vi "AppendListOfSubVIsToReport_Mutation.vi"(0 "Diagram":refnum<vi>, 5 "ObjRef":refnum<vi>, 6 "Kind":string="SubVI", 7 "Information":string="<Not A Path>") -> (3 "Replace?":bool)   [LabVIEW 2020]
uses:
  <vilib>/Utility/Data Type/NI_Data Type.lvlib
  <vilib>/Utility/Data Type/Type Definitions/Data Type.ctl
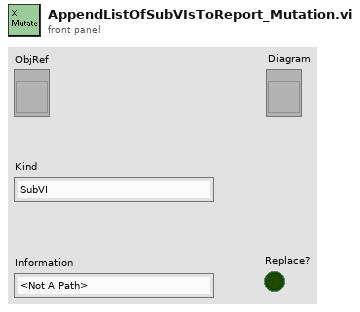
[diagram p1: front panel]
types:
  T1 = typedef "NI_Data Type.lvlib/Data Type.ctl" = enum8{"Invalid Type", "Void", "I8", "I16", "I32", "I64", "U8", "U16", "U32", "U64", "Single Float", "Double Float", "Extended Float", "Single Complex", "Double Complex", "Extended Complex", "Enum U8", "Enum U16", "Enum U32", "Enum U64", "Single Float With Unit", "Double Float With Unit", "Extended Float With Unit", "Single Complex with Unit", "Double Complex with Unit", "Extended Complex with Unit", "Boolean", "String", "Path", "Picture", "Tag", "Array", "Cluster", "Variant", "LV Variant", "Waveform", "Timestamp", "Digital Waveform", "Digital Data", "ExpressData", "Refnum", "External Data", "VI", "Poly VI", "LabVIEW Class Instance", "Fixed Point", "Set Collection", "Map Collection"}
  T2 = typedef "LVPositionTypeDef.ctl" = cluster{"Left":i32, "Top":i32}
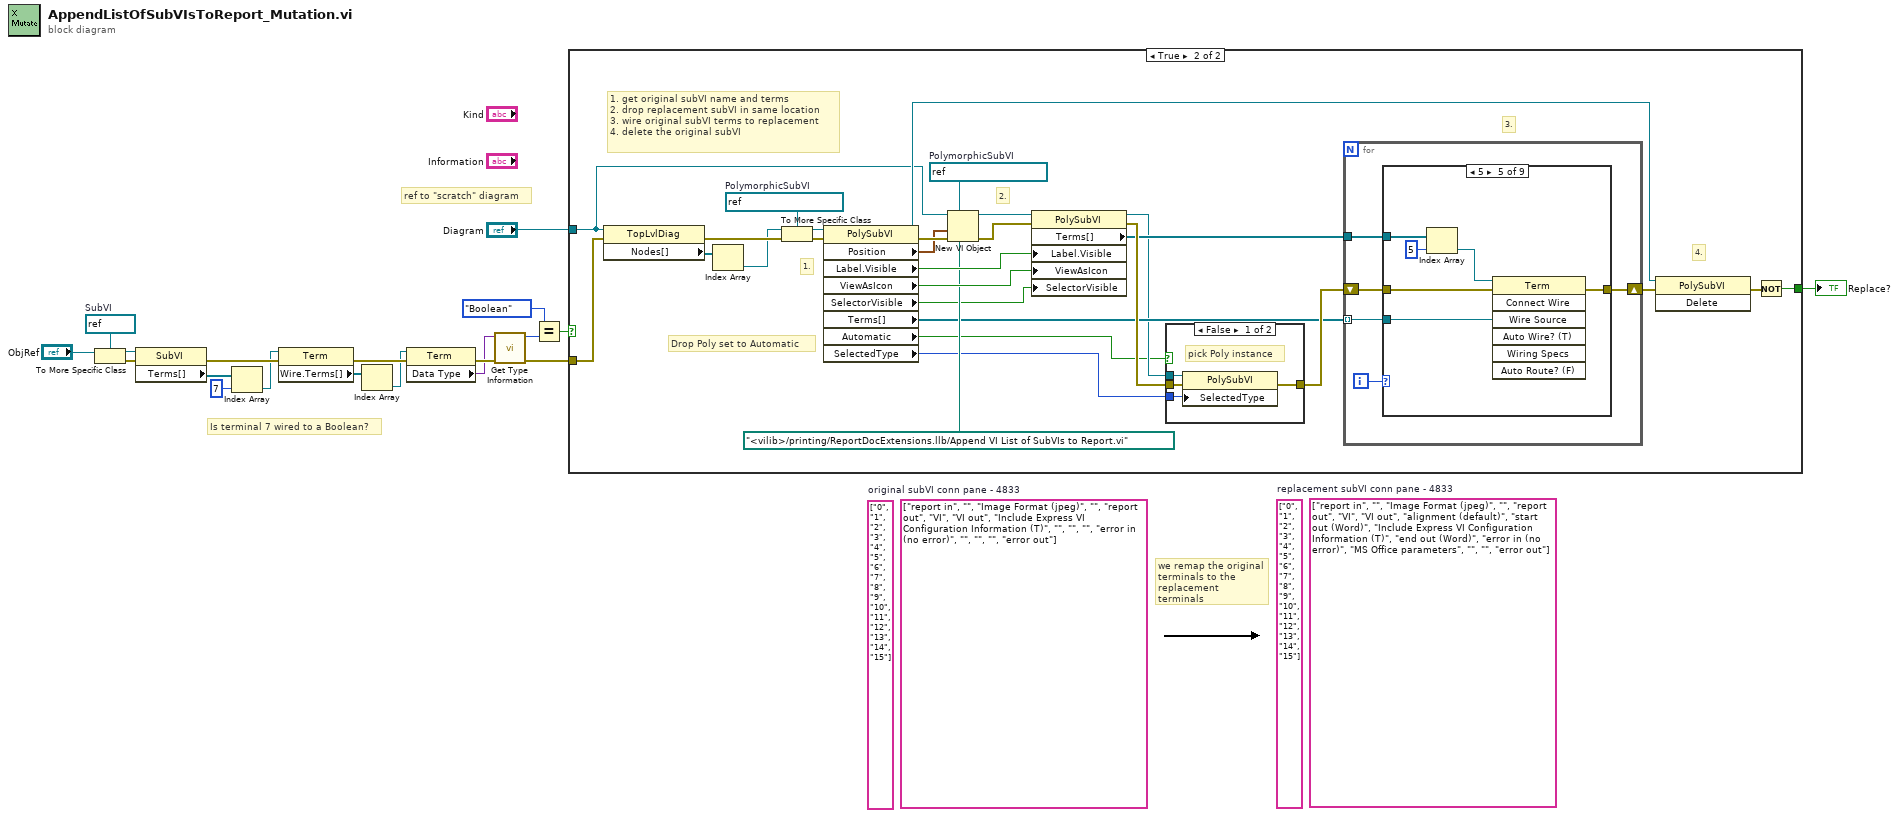
[diagram p0: block diagram]
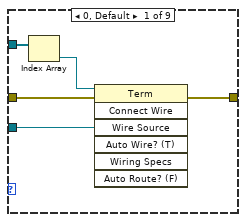
[diagram p4: hidden frame]
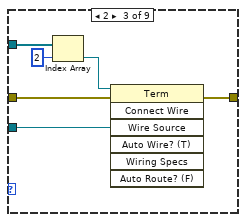
[diagram p6: hidden frame]
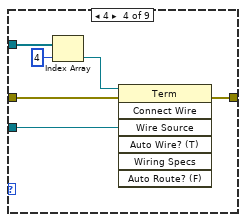
[diagram p7: hidden frame]
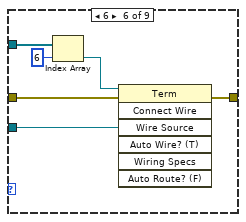
[diagram p8: hidden frame]
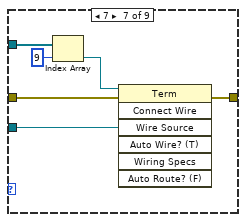
[diagram p9: hidden frame]
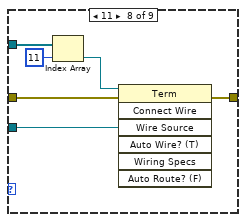
[diagram p10: hidden frame]
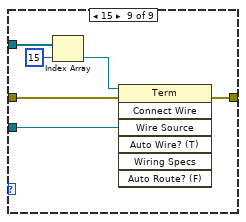
[diagram p11: hidden frame]
diagram:
  w12 = refnum<vi> refnum  # SubVI
  (unwired) string[] ["0", "1", "2", "3", "4", "5", "6", "7", "8", "9", "10", "11", "12", "13", "14", "15"]
  (unwired) string[] ["report in", "", "Image Format (jpeg)", "", "report out", "VI", "VI out", "Include Express VI Configuration Information (T)", "", "", "", "error in (no error)", "", "", "", "error out"]  # original subVI conn pane - 4833
  (unwired) string[] ["0", "1", "2", "3", "4", "5", "6", "7", "8", "9", "10", "11", "12", "13", "14", "15"]
  (unwired) string[] ["report in", "", "Image Format (jpeg)", "", "report out", "VI", "VI out", "alignment (default)", "start out (Word)", "Include Express VI Configuration Information (T)", "end out (Word)", "error in (no error)", "MS Office parameters", "", "", "error out"]  # replacement subVI conn pane - 4833
  # "Is terminal 7 wired to a Boolean?"
  # "we remap the original terminals to the replacement terminals"
  # "ref to \"scratch\" diagram"
  n1 = To More Specific Class(target class=w12, reference="ObjRef") -> (specific class reference=w10:refnum<vi>, error out=w19:errorcluster)  [unwired: 1 in]
  n2 = property class="SubVI"(reference=w10, error in=w19) -> (error out=w18:errorcluster, "Terms[]"=w9:refnum<vi>[])  [unwired: 1 out]
  n3 = Index Array(array=w9, index=7) -> (element=w7:refnum<vi>)
  n4 = property class="Term"(reference=w7, error in=w18) -> (error out=w17:errorcluster, "Wire.Terms[]"=w6:refnum<vi>[])  [unwired: 1 out]
  n5 = Index Array(array=w6) -> (element=w5:refnum<vi>)  [unwired: 1 in]
  n6 = property class="Term"(reference=w5, error in=w17) -> (error out=w16:errorcluster, "Data Type"=w4:variant)  [unwired: 1 out]
  n7 = call <vilib>:"Get Type Information.vi"("error in (no error)"=w16, "variant"=w4) -> ("error out"=w15:errorcluster, "type"=w3:T1)  [unwired: 5 in, 3 out]
  n8 = Equal?(x=Data_Type."Boolean", y=w3) -> (x = y?=w2:bool)
  n9 = case shown="True" w2 {
    tunnel: "Diagram" -> [_ w31]
    tunnel: [_ w30] -> w13
    tunnel: w15 -> [_ w41]
    frame False {
      # "If terminal 7 is not wired to a Boolean we do not need to rewire, because all the other terminals map the same."
    }
    frame True {
      w26 = refnum<vi> refnum  # PolymorphicSubVI
      w27 = refnum<vi> refnum  # PolymorphicSubVI
      # "Drop Poly set to Automatic"
      # "4."
      # "3."
      # "2."
      # "1."
      # "1. get original subVI name and terms\n2. drop replacement subVI in same location\n3. wire original subVI terms to replacement\n4. delete the original subVI"
      n10 = property class="TopLvlDiag"(reference=w31, error in=w41) -> (error out=w47:errorcluster, "Nodes[]"=w38:refnum<vi>[])  [unwired: 1 out]
      n11 = Index Array(array=w38) -> (element=w37:refnum<vi>)  [unwired: 1 in]
      n12 = To More Specific Class(target class=w27, reference=w37, error in=w47) -> (specific class reference=w32:refnum<vi>, error out=w45:errorcluster)
      n13 = property class="PolySubVI"(reference=w32, error in=w45) -> (reference out=w36:refnum<vi>, error out=w46:errorcluster, "Position"=w35:T2, "Label.Visible"=w33:bool, "ViewAsIcon"=w34:bool, "SelectorVisible"=w23:bool, "Terms[]"=w24:refnum<vi>[], "Automatic"=w21:bool, "SelectedType"=w20:i32)
      n14 = New VI Object(vi object class=w26, owner refnum=w31, position/next to=w35, 6:path "<vilib>/printing/ReportDocExtensions.llb/Append VI List of SubVIs to Report.vi", 8:w46) -> (object refnum=w28:refnum<vi>, 0:w43:errorcluster)  [unwired: 3 in]
      n15 = property class="PolySubVI"(reference=w28, error in=w43, "Label.Visible"=w33, "ViewAsIcon"=w34, "SelectorVisible"=w23) -> (reference out=w22:refnum<vi>, error out=w40:errorcluster, "Terms[]"=w29:refnum<vi>[])
      n16 = case shown="False" w21 {
        tunnel: w22 -> [w49 _]
        tunnel: w40 -> [w51 w52]
        tunnel: [w50 w52] -> w39
        tunnel: w20 -> [w48 _]
        frame False {
          # "pick Poly instance"
          n17 = property class="PolySubVI"(reference=w49, error in=w51, "SelectedType"=w48) -> (error out=w50:errorcluster)  [unwired: 1 out]
        }
        frame True {
        }
      }
      n18 = for {
        tunnel: w24 -> [w54] mode=indexing
        tunnel: w29 -> [w53]
        shift-right: [w56] -> w44
        shift-left: w39 -> [w57]
        i -> [w55]
        n19 = case shown="5" w55 {
          tunnel: w54 -> [w60 _ w67 w73 w79 w85 w91 w97 w103]
          tunnel: w53 -> [w59 _ w66 w72 w78 w84 w90 w96 w102]
          tunnel: w57 -> [w62 w63 w69 w75 w81 w87 w93 w99 w105]
          tunnel: [w61 w63 w68 w74 w80 w86 w92 w98 w104] -> w56
          frame 0, Default {
            n20 = Index Array(array=w59) -> (element=w58:refnum<vi>)  [unwired: 1 in]
            n21 = invoke class="Term" method="Connect Wire"(reference=w58, error in=w62, "Wire Source"=w60) -> (error out=w61:errorcluster)  [unwired: 4 in, 6 out]
          }
          frame 1, 3, 8..10, 12..14 {
          }
          frame 2 {
            n22 = Index Array(array=w66, index=2) -> (element=w64:refnum<vi>)
            n23 = invoke class="Term" method="Connect Wire"(reference=w64, error in=w69, "Wire Source"=w67) -> (error out=w68:errorcluster)  [unwired: 4 in, 6 out]
          }
          frame 4 {
            n24 = Index Array(array=w72, index=4) -> (element=w70:refnum<vi>)
            n25 = invoke class="Term" method="Connect Wire"(reference=w70, error in=w75, "Wire Source"=w73) -> (error out=w74:errorcluster)  [unwired: 4 in, 6 out]
          }
          frame 5 {
            n26 = Index Array(array=w78, index=5) -> (element=w76:refnum<vi>)
            n27 = invoke class="Term" method="Connect Wire"(reference=w76, error in=w81, "Wire Source"=w79) -> (error out=w80:errorcluster)  [unwired: 4 in, 6 out]
          }
          frame 6 {
            n28 = Index Array(array=w84, index=6) -> (element=w82:refnum<vi>)
            n29 = invoke class="Term" method="Connect Wire"(reference=w82, error in=w87, "Wire Source"=w85) -> (error out=w86:errorcluster)  [unwired: 4 in, 6 out]
          }
          frame 7 {
            n30 = Index Array(array=w90, index=9) -> (element=w88:refnum<vi>)
            n31 = invoke class="Term" method="Connect Wire"(reference=w88, error in=w93, "Wire Source"=w91) -> (error out=w92:errorcluster)  [unwired: 4 in, 6 out]
          }
          frame 11 {
            n32 = Index Array(array=w96, index=11) -> (element=w94:refnum<vi>)
            n33 = invoke class="Term" method="Connect Wire"(reference=w94, error in=w99, "Wire Source"=w97) -> (error out=w98:errorcluster)  [unwired: 4 in, 6 out]
          }
          frame 15 {
            n34 = Index Array(array=w102, index=15) -> (element=w100:refnum<vi>)
            n35 = invoke class="Term" method="Connect Wire"(reference=w100, error in=w105, "Wire Source"=w103) -> (error out=w104:errorcluster)  [unwired: 4 in, 6 out]
          }
        }
      }
      n36 = invoke class="PolySubVI" method="Delete"(reference=w36, error in=w44) -> (error out=w42:errorcluster)  [unwired: 1 in, 2 out]
      n37 = Not(x=w42) -> (.not. x?=w30:bool)
    }
  }
  "Replace?" <- w13
